vi "Test-Sgraph-system.vi"() -> ()   [LabVIEW 2020]
uses:
  <vilib>/Platform/TimedLoop/XDataNode/timing_clust.ctl
  <vilib>/Platform/TimedLoop/XDataNode/nitl_modes.ctl
  <vilib>/Platform/TimedLoop/XDataNode/wakeup.ctl
  Common/controls/Global-services.vi
  <vilib>/platform/TimedLoop/XDataNode/XDataNode.xnode
  <vilib>/Platform/TimedLoop/XDataNode/XDNodeRunTimeDep.lvlib
  Gserver/Gserver.lvclass
  HISW/HISW.lvclass
panel:
  in  "OpenGraph":bool caption="Graph"
  out "Numeric 2":i32
  out "HMI-error":bool
  out "Numeric":i32
  in  "Gserver":bool
  in  "FAMM":bool
  in  "HISW":bool
  in  "Stop DAQ":bool
  out "DAQ":picture
  in  "DAQ":bool
  # "Test Sgraph data historian test utility"
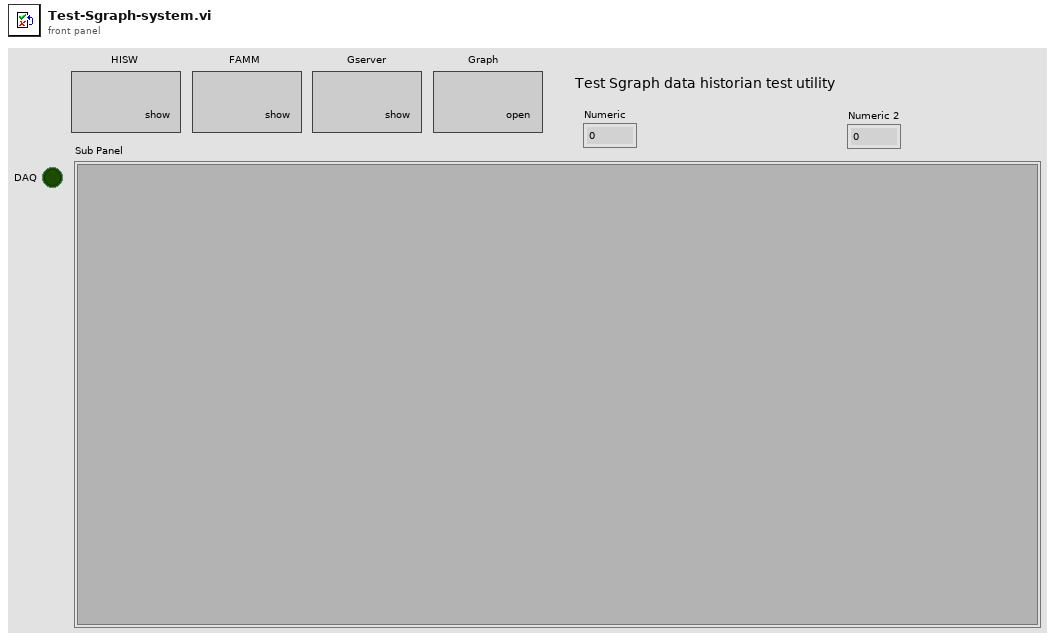
[diagram p1: front panel]
types:
  T1 = typedef "XDNodeRunTimeDep.lvlib/timing_clust.ctl" = cluster{"Expected End [f-1]":u64, "Actual End [f-1]":u64, "Finished Late? [f-1]":bool, "Expected End [i-1]":u64, "Actual End [i-1]":u64, "Finished Late? [i-1]":bool, "Expected Start [i]":u64, "Actual Start [i]":u64, "Expected Start [f]":u64, "Actual Start [f]":u64, "Source Name":string, "Structure Name":string, "Period":i64, "Deadline":i64, "Offset":i64, "Start":i64, "Priority":i32, "Timeout":i32, "Mode":T2, "Wakeup Reason":T3, "Error":errorcluster, "Source Type":string, "Secondary Source Type":string, "Global End Time":u64, "Global Start Time":u64, "Frame Duration":u64, "Iteration Duration":u64, "Assigned CPU":i32, "I/O Scan Engine Mode":u32}
  T2 = typedef "XDNodeRunTimeDep.lvlib/nitl_modes.ctl" = enum32{"No Change", "Process missed periods, maintain original phase", "Discard missed periods, maintain original phase", "Process missed periods, ignore original phase", "Discard missed periods, ignore original phase"}
  T3 = typedef "XDNodeRunTimeDep.lvlib/wakeup.ctl" = enum32{"Normal", "Aborted", "Asynchronous wakeup", "Timing source error", "Timed loop error", "Timeout"}
  T4 = typedef "typedef_PAQsample.ctl" = cluster{"Time Stamp":timestamp, "TAGs":string[], "status":u32[], "data":dbl[], "Source":string}
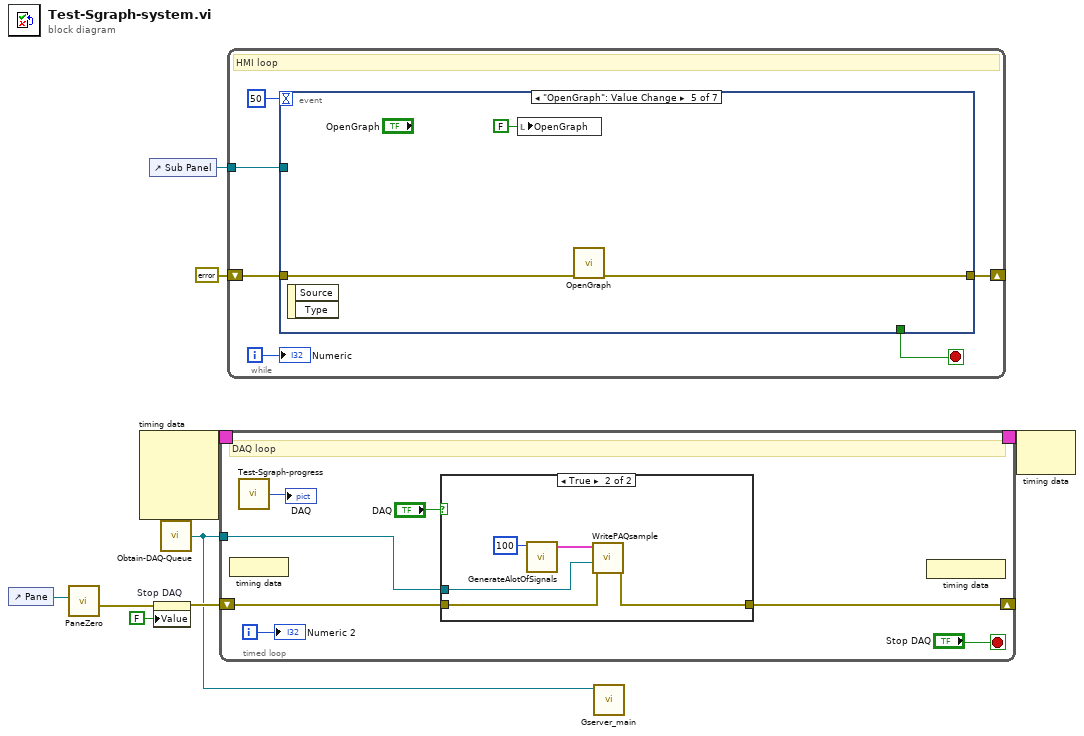
[diagram p0: block diagram]
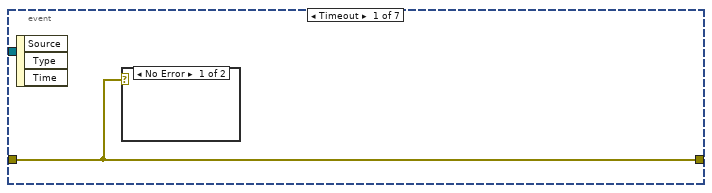
[diagram p3: hidden frame]
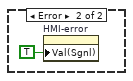
[diagram p4: hidden frame]
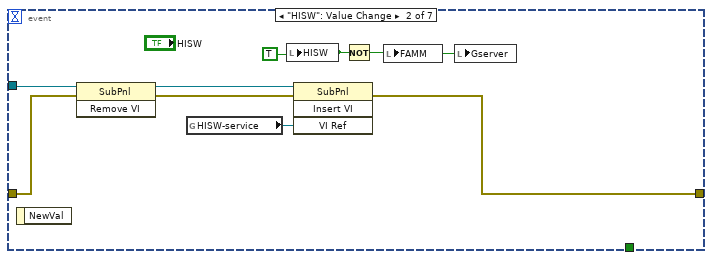
[diagram p5: hidden frame]
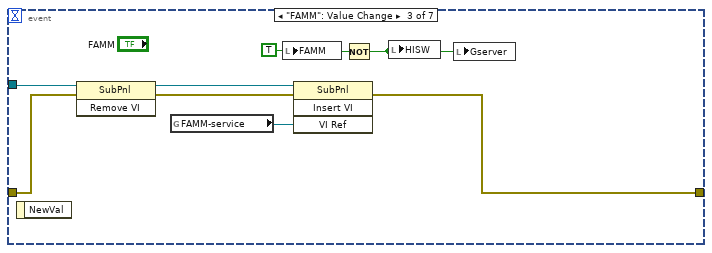
[diagram p6: hidden frame]
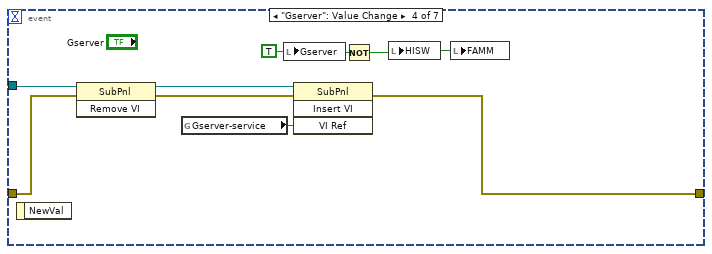
[diagram p7: hidden frame]
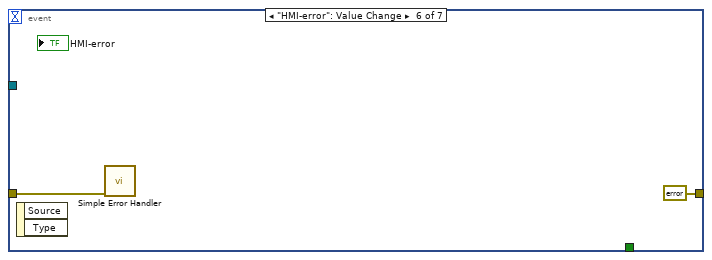
[diagram p8: hidden frame]
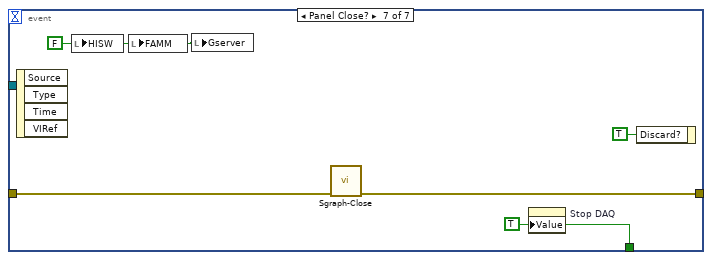
[diagram p9: hidden frame]
diagram:
  n1 = control-ref of="Pane"() -> (w2:refnum<vi>)
  n2 = call "PaneZero.vi"("Pane"=w2) -> ("error out"=w3:errorcluster)  [unwired: 10 in]
  n3 = node-c288() -> (w9:T1)  [unwired: 4 in]
  n4 = control-ref of="Sub Panel"() -> (w5:refnum<vi>)
  n5 = property on="Stop DAQ" class="Bool (strict)"(error in=w3, "Value"=FALSE ("Stop DAQ")) -> (error out=w6:errorcluster)  [unwired: 1 in, 1 out]
  n6 = call "Obtain-DAQ-Queue.vi"() -> ("DAQ-Queue"=w1:refnum<queue>)  [unwired: 7 in]
  n7 = timed-loop {
    timing: w9 -> [_]
    timing-out: [_] -> w8
    shift-right: [w12] -> _
    shift-left: w6 -> [w13]
    tunnel: w1 -> [w10]
    i -> [w11]
    stop <- "Stop DAQ" stop-if-true
    # "DAQ loop"
    n8 = node-c288() -> ()  [unwired: 1 in]
    n9 = call "Test-Sgraph-progress.vi"() -> ("37x37"=→"DAQ":picture)  [unwired: 7 in]
    n10 = case shown="True" "DAQ" {
      tunnel: w13 -> [w17 w20]
      tunnel: [w17 w19] -> w12
      tunnel: w10 -> [_ w18]
      frame False {
      }
      frame True {
        n11 = call "GenerateAlotOfSignals.vi"("Channels"=100) -> ("DAQ"=w21:T4)  [unwired: 10 in]
        n12 = call "WritePAQsample.vi"("error in (no error)"=w20, "DAQ-Queue"=w18, "PAQ IN"=w21) -> ("error out"=w19:errorcluster)  [unwired: 7 in, 1 out]
      }
    }
    n13 = node-c288() -> ()  [unwired: 1 out]
    "Numeric 2" <- w11
  }
  n14 = while {
    tunnel: w5 -> [w29]
    shift-right: [w28] -> _
    shift-left: errorcluster {"status"=FALSE, "code"=0, "source"=""} ("error out") -> [w27]
    i -> [w25]
    stop <- w26 stop-if-true
    # "HMI loop"
    n15 = event shown="[4] \"OpenGraph\": Value Change" {
      selector: _ -> [_ _ _ _ _ _ _]
      dyn-events: _ -> [_ _ _ _ _ _ _]
      timeout: 50 -> [_ _ _ _ _ _ _]
      tunnel: [_ _ _ _ _ _ w65] -> w26
      tunnel: w29 -> [_ w38 w48 w56 _ _ _]
      tunnel: [w31 w34 w44 w52 w58 errorcluster {"status"=FALSE, "code"=0, "source"=""} ("error out") w63] -> w28
      tunnel: w27 -> [w31 w33 w43 w51 w57 w60 w64]
      event Timeout {
        n16 = event-data() -> ()  [unwired: 1 in, 3 out]
        n17 = case shown="No Error" w31 {
          frame No Error {
          }
          frame Error {
            n18 = property on="HMI-error" class="Bool (strict)"("Val(Sgnl)"=TRUE ("Value (Signaling)")) -> ()  [unwired: 2 in, 2 out]
          }
        }
      }
      event "HISW": Value Change {
        w40 = TRUE ("HISW")
        n19 = event-data() -> ()  [unwired: 1 in, 1 out]
        n20 = invoke class="SubPnl" method="Remove VI"(reference=w38, error in=w33) -> (reference out=w37:refnum<vi>, error out=w35:errorcluster)  [unwired: 1 in, 1 out]
        n21 = global read "Global-services.vi" "HISW-service"() -> (w36:refnum<vi>)
        n22 = local write "HISW"(w40) -> ()
        n23 = invoke class="SubPnl" method="Insert VI"(reference=w37, error in=w35, "VI Ref"=w36) -> (error out=w34:errorcluster)  [unwired: 1 in, 3 out]
        n24 = Not(x=w40) -> (.not. x?=w39:bool)
        n25 = local write "FAMM"(w39) -> ()
        n26 = local write "Gserver"(w39) -> ()
      }
      event "FAMM": Value Change {
        w42 = TRUE ("HISW")
        n27 = event-data() -> ()  [unwired: 1 in, 1 out]
        n28 = invoke class="SubPnl" method="Remove VI"(reference=w48, error in=w43) -> (reference out=w47:refnum<vi>, error out=w45:errorcluster)  [unwired: 1 in, 1 out]
        n29 = global read "Global-services.vi" "FAMM-service"() -> (w46:refnum<vi>)
        n30 = local write "FAMM"(w42) -> ()
        n31 = invoke class="SubPnl" method="Insert VI"(reference=w47, error in=w45, "VI Ref"=w46) -> (error out=w44:errorcluster)  [unwired: 1 in, 3 out]
        n32 = Not(x=w42) -> (.not. x?=w41:bool)
        n33 = local write "HISW"(w41) -> ()
        n34 = local write "Gserver"(w41) -> ()
      }
      event "Gserver": Value Change {
        w50 = TRUE ("HISW")
        n35 = event-data() -> ()  [unwired: 1 in, 1 out]
        n36 = invoke class="SubPnl" method="Remove VI"(reference=w56, error in=w51) -> (reference out=w55:refnum<vi>, error out=w53:errorcluster)  [unwired: 1 in, 1 out]
        n37 = global read "Global-services.vi" "Gserver-service"() -> (w54:refnum<vi>)
        n38 = local write "Gserver"(w50) -> ()
        n39 = invoke class="SubPnl" method="Insert VI"(reference=w55, error in=w53, "VI Ref"=w54) -> (error out=w52:errorcluster)  [unwired: 1 in, 3 out]
        n40 = Not(x=w50) -> (.not. x?=w49:bool)
        n41 = local write "HISW"(w49) -> ()
        n42 = local write "FAMM"(w49) -> ()
      }
      event "OpenGraph": Value Change {
        n43 = event-data() -> ()  [unwired: 1 in, 2 out]
        n44 = local write "OpenGraph"(FALSE ("OpenGraph")) -> ()
        n45 = call "OpenGraph.vi"("error in (no error)"=w57) -> ("Error out"=w58:errorcluster)  [unwired: 10 in]
      }
      event "HMI-error": Value Change {
        n46 = event-data() -> ()  [unwired: 1 in, 2 out]
        n47 = call <vilib>:"Simple Error Handler.vi"("error in (no error)"=w60) -> ()  [unwired: 4 in, 5 out]
      }
      event Panel Close? {
        w62 = FALSE ("HISW")
        w65 = TRUE ("Stop DAQ")
        n48 = event-data() -> ()  [unwired: 1 in, 4 out]
        n49 = local write "HISW"(w62) -> ()
        n50 = local write "FAMM"(w62) -> ()
        n51 = local write "Gserver"(w62) -> ()
        n52 = call "Sgraph-Close.vi"("error in (no error)"=w64) -> ("error out"=w63:errorcluster)  [unwired: 10 in]
        n53 = property on="Stop DAQ" class="Bool (strict)"("Value"=w65) -> ()  [unwired: 2 in, 2 out]
        n54 = event-data("Discard?"=TRUE) -> ()  [unwired: 1 in, 1 out]
      }
    }
    "Numeric" <- w25
  }
  n55 = call "Gserver_main.vi"("DAQ-Queue"=w1) -> ()  [unwired: 11 in]
  n56 = node-c288(w8) -> ()  [unwired: 1 out]
